vi "KB-活动单元格触发.vi"(11 "Data Result":refnum<vi>) -> ()   [LabVIEW 2015]
uses:
  <vilib>/Utility/miscctls.llb/LVRowAndColumnTypeDef.ctl
panel:
  in  "Data Result 2":string[][](table)
  out "数值":i32
  out "子数组":string[](array[string])
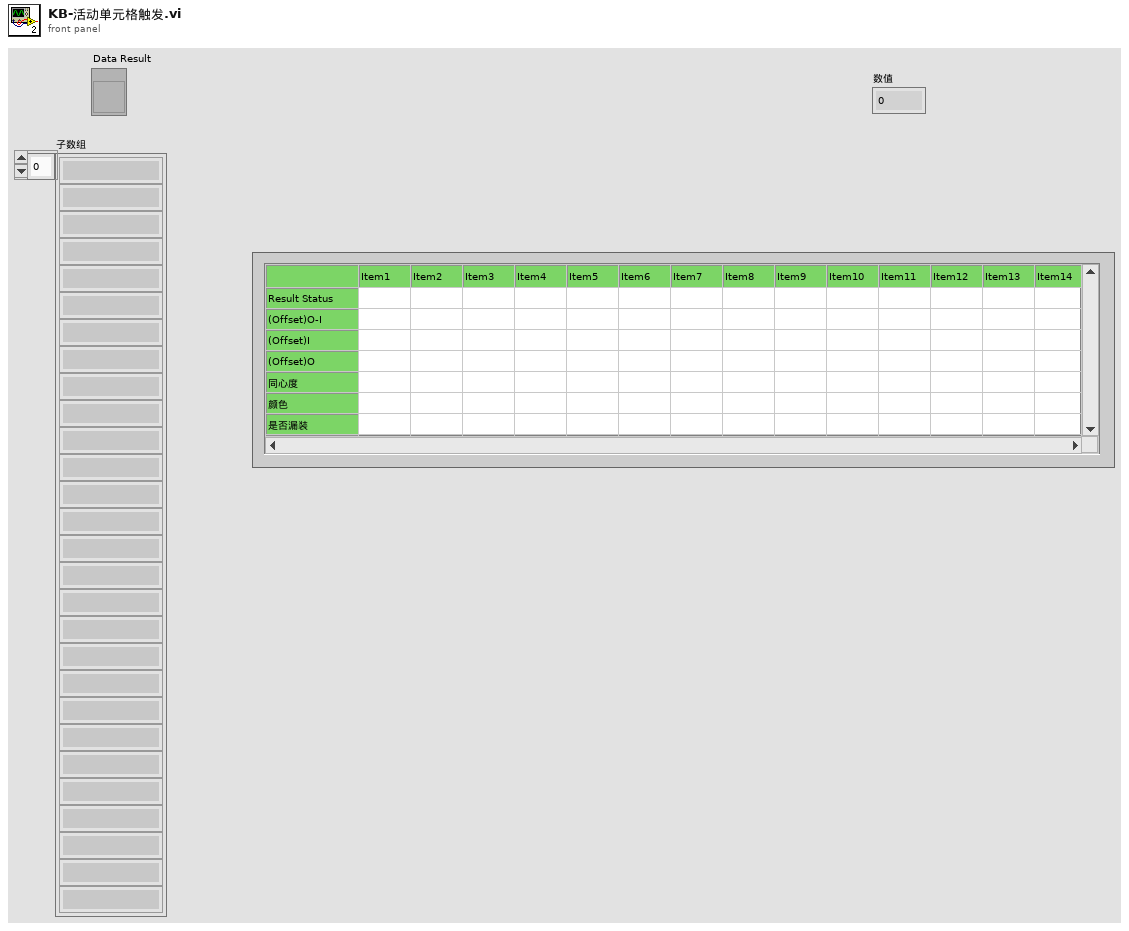
[diagram p1: front panel]
types:
  T1 = typedef "LVRowAndColumnTypeDef.ctl" = cluster{"Row":i32, "Column":i32}
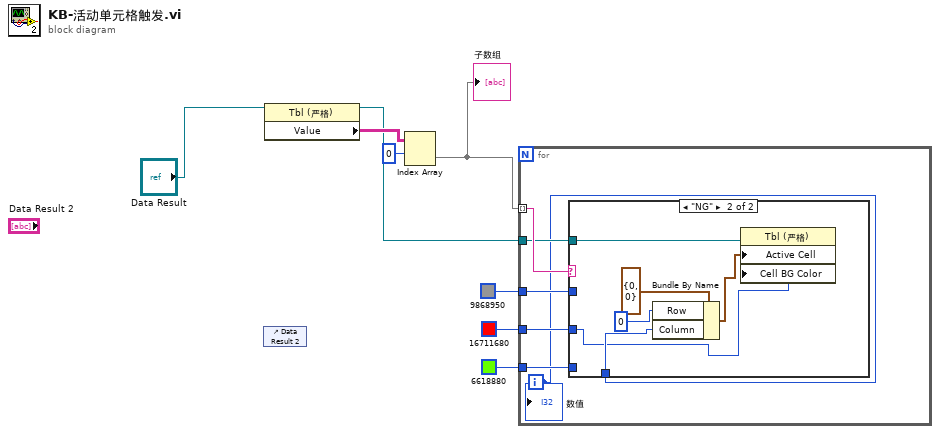
[diagram p0: block diagram]
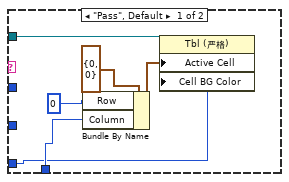
[diagram p2: hidden frame]
diagram:
  n1 = control-ref of="Data Result 2"() -> ()  [unwired: 1 out]
  n2 = property class="Tbl (严格)"(reference="Data Result") -> (reference out=w1:refnum<vi>, "Value"=w2:string[][])  [unwired: 1 in, 1 out]
  n3 = Index Array(array=w2, index (row)=0 ("索引 (行)")) -> (element=w7:string[])  [unwired: 1 in]
  "子数组" <- w7
  n4 = for {
    tunnel: w7 -> [w14] mode=indexing
    tunnel: w1 -> [w13]
    tunnel: u32 9868950 -> [w12]
    tunnel: u32 16711680 -> [w11]
    tunnel: u32 6618880 -> [w10]
    i -> [w9]
    n5 = case shown="\"NG\"" w14 {
      tunnel: w13 -> [w20 w26]
      tunnel: w12 -> [_ _]
      tunnel: w11 -> [_ w21]
      tunnel: w9 -> [w17 w23]
      tunnel: w10 -> [w15 _]
      frame "Pass", Default {
        n6 = Bundle By Name(cluster=T1 {"Row"=0, "Column"=0} ("活动单元格:活动单元格"), "Row"=0, "Column"=w17) -> (w16:T1)
        n7 = property class="Tbl (严格)"(reference=w20, "Active Cell"=w16, "Cell BG Color"=w15) -> ()  [unwired: 1 in, 2 out]
      }
      frame "NG" {
        n8 = Bundle By Name(cluster=T1 {"Row"=0, "Column"=0} ("选择区域起始"), "Row"=0, "Column"=w23) -> (w22:T1)
        n9 = property class="Tbl (严格)"(reference=w26, "Active Cell"=w22, "Cell BG Color"=w21) -> ()  [unwired: 1 in, 2 out]
      }
    }
    "数值" <- w9
  }
